vi "EditShape Response.vi"(8 "error in (no error)":errorcluster, 10 "Shape Reference":refnum<data-value>, 11 "Editor Handler in":refnum<class "Image Editor Handler.lvclass">) -> (0 "error out":errorcluster, 3 "Editor Handler out":refnum<class "Image Editor Handler.lvclass">)   [LabVIEW 2017, in "LV Image Editor Framework.lvlib" / "Image Editor Handler.lvclass"]
uses:
  <vilib>/LIEF/Image Editor Handler/Image Editor Handler.lvclass
  <vilib>/LIEF/Forms/Shape/Shape.lvclass
  <vilib>/LIEF/Image Editor Handler/Image Editor Handler.lvclass/Image Editor Handler.ctl
  <vilib>/LIEF/Image/Image.lvclass
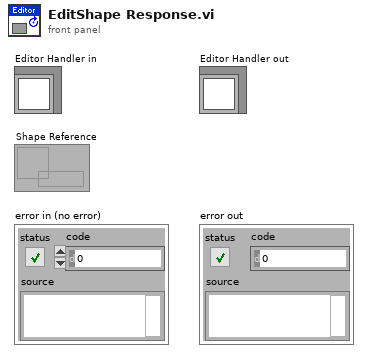
[diagram p1: front panel]
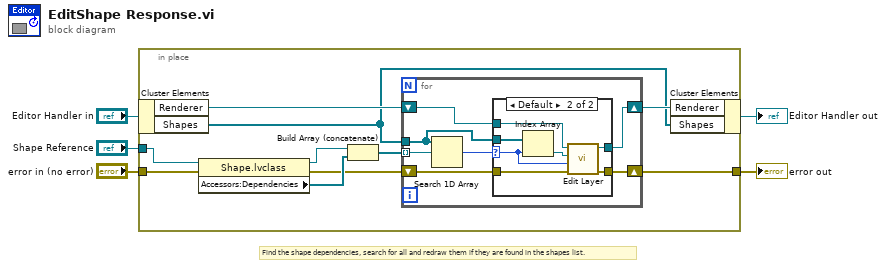
[diagram p0: block diagram]
diagram:
  # "Find the shape dependencies, search for all and redraw them if they are found in the shapes list."
  n1 = in-place {
    in-place-border: "Shape Reference" -> [w10]
    in-place-border: "error in (no error)" -> [w8]
    in-place-border: [w12] -> w5
    n2 = in-place-cluster #1("Editor Handler in") -> ("Renderer"=w15:refnum<class "Image.lvclass">, "Shapes"=w13:refnum<data-value>[])
    n3 = property class="Shape.lvclass"(reference=w10, error in=w8) -> (reference out=w6:refnum<data-value>, error out=w7:errorcluster, "Accessors:Dependencies"=w11:refnum<data-value>[])
    n4 = Build Array (concatenate)(w6, w11) -> (w9:refnum<data-value>[])
    n5 = for {
      tunnel: w13 -> [w20]
      shift-right: [w21] -> w14
      shift-left: w15 -> [w22]
      shift-right: [w18] -> w12
      shift-left: w7 -> [w19]
      tunnel: w9 -> [w17] mode=indexing
      n6 = Search 1D Array(1D array=w20, element=w17) -> (index of element=w16:i32)  [unwired: 1 in]
      n7 = case shown="Default" w16 {
        selector: w16 -> [_ w25]
        tunnel: w22 -> [w24 w31]
        tunnel: [w24 w30] -> w21
        tunnel: w20 -> [_ w28]
        tunnel: w19 -> [w23 w27]
        tunnel: [w23 w26] -> w18
        frame -1 {
        }
        frame Default {
          n8 = Index Array(array=w28, index=w25) -> (element=w29:refnum<data-value>)
          n9 = call <vilib>:"Edit Layer.vi"("error in (no error)"=w27, "Layer Index"=w25, "ShapeRef"=w29, "Image in"=w31) -> ("error out"=w26:errorcluster, "Image out"=w30:refnum<class "Image.lvclass">)  [unwired: 6 in]
        }
      }
    }
    n10 = in-place-cluster #1("Renderer"=w14, "Shapes"=w13) -> (→"Editor Handler out":refnum<class "Image Editor Handler.lvclass">)
  }
  "error out" <- w5
